vi "VI Controls.vi"   [LabVIEW 2025]
doc: "Author: Scott Hannahs <sth@magnet.fsu.edu>\n\nThis software is licensed for use under the “MIT License\"\nCopyright (c) 2025 Scott Hannahs, sth@sth@magnet.sthnet.net\n\nPermission is hereby granted, free of charge, to any person obtaining a copy of this software and associated documentation files (the \"Software\"), to deal in the Software without restriction, including without limitation the rights to use, copy, modify, merge, publish, distribute, sublicense, and/or sell copies of the Software, and to permit persons to whom the Software is furnished to do so, subject to the following conditions: The above copyright notice and this permission notice shall be included in all copies or substantial portions of the Software.\n\nTHE SOFTWARE IS PROVIDED \"AS IS\", WITHOUT WARRANTY OF ANY KIND, EXPRESS OR IMPLIED, INCLUDING BUT NOT LIMITED TO THE WARRANTIES OF MERCHANTABILITY, FITNESS FOR A PARTICULAR PURPOSE AND NONINFRINGEMENT. IN NO EVENT SHALL THE AUTHORS OR COPYRIGHT HOLDERS BE LIABLE FOR ANY CLAIM, DAMAGES OR OTHER LIABILITY, WHETHER IN AN ACTION OF CONTRACT, TORT OR OTHERWISE, ARISING FROM, OUT OF OR IN CONNECTION WITH THE SOFTWARE OR THE USE OR OTHER DEALINGS IN THE SOFTWARE."
uses:
  <vilib>/Utility/victl.llb/VIParam.ctl
  <vilib>/Utility/file.llb/Read From Spreadsheet File (DBL).vi
types:
  T1 = typedef "VIParam.ctl" = cluster{"control\nname":string, "type\ndescriptor":i16[], "flattened\ndata":string}[]
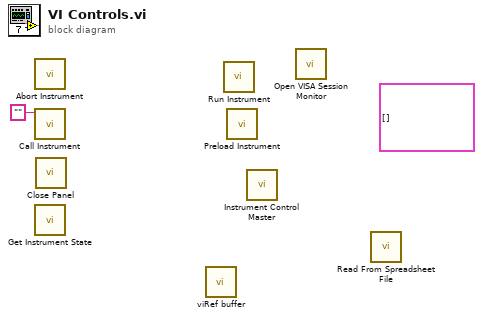
[diagram p0: block diagram]
diagram:
  (unwired) T1 [] ("Inputs [{name, type, data}]")
  n1 = call <vilib>:"Abort Instrument.vi"() -> ()  [unwired: 11 in, 1 out]
  n2 = call <vilib>:"Call Instrument.vi"("VI name"="") -> ()  [unwired: 9 in, 2 out]
  n3 = call <vilib>:"Get Instrument State.vi"() -> ()  [unwired: 9 in, 3 out]
  n4 = call <vilib>:"Close Panel.vi"() -> ()  [unwired: 11 in, 1 out]
  n5 = call <vilib>:"viRef buffer.vi"() -> ()  [unwired: 6 in, 2 out]
  n6 = call <vilib>:"Run Instrument.vi"() -> ()  [unwired: 11 in, 1 out]
  n7 = call <vilib>:"Preload Instrument.vi"() -> ()  [unwired: 11 in, 1 out]
  n8 = call <vilib>:"Instrument Control Master.vi"() -> ()  [unwired: 15 in, 5 out]
  n9 = call <vilib>:"Open VISA Session Monitor.vi"() -> ()  [unwired: 1 in]
  n10 = call-poly <vilib>:"Read From Spreadsheet File.vi"() -> ()  [unwired: 7 in, 5 out]
